vi "RT Main.vi"() -> ()   [LabVIEW 2018]
doc: "The myRIO Custom FPGA Project template acquires button data from the onboard button and displays the button value on a Boolean indicator. The SYS.RDY indicator shows the FPGA status."
uses:
  <vilib>/Stratom, Inc/X-CAN for myRIO (API)/X-CAN Class/Type Definitions/CANFrame.ctl
  <vilib>/Stratom, Inc/X-Modules for myRIO/Type Defs/MXPChannel.ctl
  <vilib>/Stratom, Inc/X-CAN for myRIO (API)/X-CAN Class/Type Definitions/CAN_Speed.ctl
  <vilib>/Platform/TimedLoop/XDataNode/timing_clust.ctl
  <vilib>/Platform/TimedLoop/XDataNode/nitl_modes.ctl
  <vilib>/Platform/TimedLoop/XDataNode/wakeup.ctl
  <vilib>/myRIO/Instrument Drivers/Onboard IO/I2C/typedefs/I2C User Configuration.ctl
  <vilib>/myRIO/Instrument Drivers/Onboard IO/I2C/typedefs/I2C Transfer Rate.ctl
  <vilib>/myRIO/Instrument Drivers/Onboard IO/I2C/typedefs/I2C Reference.ctl
  <vilib>/myRIO/Common/Instrument Driver Framework/Utilities/typedefs/myRIO Generic Hardware Reference.ctl
  <vilib>/myRIO/Common/Instrument Driver Framework/Utilities/typedefs/Hardware Version Enum.ctl
  <vilib>/myRIO/Common/Instrument Driver Framework/Utilities/typedefs/myRIO v1.0 Reference.ctl
  <vilib>/myRIO/Common/Instrument Driver Framework/Utilities/typedefs/Generic FPGA Reference.ctl
  <vilib>/myRIO/Common/Instrument Driver Framework/myRIO v1.0/I2C/typedefs/I2C Channels Enum.ctl
  <vilib>/myRIO/Instrument Drivers/Onboard IO/I2C/typedefs/I2C Configuration.ctl
  <vilib>/userdefined/High Color/nirio_resource_hc.ctl
  <vilib>/myRIO/Instrument Drivers/Onboard IO/AI/typedefs/AI Reference.ctl
  <vilib>/myRIO/Common/Instrument Driver Framework/myRIO v1.0/AI/typedefs/AI Channels List.ctl
  <vilib>/myRIO/Common/Instrument Driver Framework/myRIO v1.0/AI/typedefs/AI Channels Enum.ctl
  <vilib>/myRIO/Common/Instrument Driver Framework/Utilities/typedefs/Analog Scaling Constants List.ctl
  <vilib>/myRIO/Common/Instrument Driver Framework/Utilities/typedefs/Analog Scaling Constants.ctl
  <vilib>/myRIO/Instrument Drivers/Onboard IO/DIO/typedefs/DIO Reference.ctl
  <vilib>/myRIO/Common/Instrument Driver Framework/myRIO v1.0/DIO/typedefs/DIO Channels List.ctl
  <vilib>/myRIO/Common/Instrument Driver Framework/myRIO v1.0/DIO/typedefs/DIO Channels Enum.ctl
  <vilib>/imath/engines/lvmath/Plug In/_Char/NIMS_CH_character datatype.ctl
  <vilib>/myRIO/Instrument Drivers/Onboard IO/AO/typedefs/AO Reference.ctl
  <vilib>/myRIO/Common/Instrument Driver Framework/myRIO v1.0/AO/typedefs/AO Channels List.ctl
  <vilib>/myRIO/Common/Instrument Driver Framework/myRIO v1.0/AO/typedefs/AO Channels Enum.ctl
  <vilib>/myRIO/Common/Instrument Driver Framework/Utilities/vis/Is FPGA Ref Available.vi
  <vilib>/myRIO/Common/Instrument Driver Framework/myRIO v1.0/I2C/vis/myRIO v1.1 Open I2C.vi
  <vilib>/myRIO/Instrument Drivers/Onboard IO/I2C/vis/Configure.vi
  <vilib>/myRIO/Instrument Drivers/Onboard IO/I2C/vis/Write Read.vi
  <vilib>/myRIO/Common/Instrument Driver Framework/myRIO v1.0/AI/vis/myRIO v1.1 Open AI.vi
  <vilib>/myRIO/Instrument Drivers/Onboard IO/AI/vis/Read.vi
  <vilib>/myRIO/Common/Instrument Driver Framework/myRIO v1.0/DIO/vis/myRIO v1.1 Open DIO.vi
  <vilib>/myRIO/Instrument Drivers/Onboard IO/DIO/vis/Write.vi
  <vilib>/myRIO/Common/Instrument Driver Framework/myRIO v1.0/AO/vis/myRIO v1.1 Open AO.vi
  <vilib>/myRIO/Instrument Drivers/Onboard IO/AO/vis/Write.vi
  <vilib>/myRIO/Instrument Drivers/Onboard IO/DIO/vis/Read.vi
  <vilib>/myRIO/Common/Instrument Driver Framework/Utilities/vis/Validate Channels.vi
  <vilib>/myRIO/Common/Instrument Driver Framework/myRIO v1.0/I2C/vis/myRIO v1.0 Reserve I2C.vi
  <vilib>/myRIO/Common/Instrument Driver Framework/myRIO v1.0/AI/vis/myRIO v1.0 Reserve AI.vi
  <vilib>/myRIO/Common/Instrument Driver Framework/myRIO v1.0/DIO/vis/myRIO v1.0 Reserve DIO.vi
  <vilib>/myRIO/Common/Instrument Driver Framework/myRIO v1.0/AO/vis/myRIO v1.0 Reserve AO.vi
  <vilib>/myRIO/Common/Instrument Driver Framework/myRIO v1.0/I2C/vis/myRIO v1.0 Build MUX Configuration I2C.vi
  <vilib>/myRIO/Common/Instrument Driver Framework/myRIO v1.0/Resource Manager/vis/myRIO v1.0 Reserve Channel List.vi
  <vilib>/myRIO/Common/Instrument Driver Framework/myRIO v1.0/AI/vis/myRIO v1.0 Build MUX Configuration AI.vi
  <vilib>/myRIO/Common/Instrument Driver Framework/myRIO v1.0/DIO/vis/myRIO v1.0 Build MUX Configuration DIO.vi
  <vilib>/myRIO/Common/Instrument Driver Framework/myRIO v1.0/AO/vis/myRIO v1.0 Build MUX Configuration AO.vi
  <vilib>/myRIO/Common/Instrument Driver Framework/myRIO v1.0/Resource Manager/vis/myRIO v1.0 Create Configuration List.vi
  <vilib>/myRIO/Common/Instrument Driver Framework/myRIO v1.0/Resource Manager/vis/myRIO v1.0 Reserve Channel.vi
  <vilib>/myRIO/Common/Instrument Driver Framework/myRIO v1.0/Resource Manager/vis/myRIO v1.0 Unreserve Channel.vi
  <vilib>/myRIO/Common/Instrument Driver Framework/myRIO v1.0/Resource Manager/vis/myRIO v1.0 Build Mutex Name.vi
  <vilib>/functionblocks/Counter/Pulse Timer/Pulse Timer.vi
  <vilib>/Utility/VariantDataType/GetNumericInfo.vi
  <vilib>/Utility/error.llb/Error Cluster From Error Code.vi
  <vilib>/myRIO/Common/Instrument Driver Framework/myRIO v1.0/myRIO v1.1 Open.vi
  <vilib>/myRIO/Common/Instrument Driver Framework/Utilities/vis/IO Manager.vi
  <vilib>/myRIO/Common/Instrument Driver Framework/Utilities/vis/Configuration Manager.vi
  <vilib>/myRIO/Common/Instrument Driver Framework/myRIO v1.0/Resource Manager/vis/myRIO v1.0 Configure IO.vi
  <vilib>/myRIO/Common/Instrument Driver Framework/myRIO v1.0/myRIO v1.0 Close.vi
  <vilib>/myRIO/Common/Instrument Driver Framework/myRIO v1.0/DIO/vis/myRIO v1.0 Read DIO.vi
  <vilib>/myRIO/Common/Instrument Driver Framework/myRIO v1.0/DIO/vis/myRIO v1.0 Write DIO.vi
  <vilib>/myRIO/Common/Instrument Driver Framework/myRIO v1.0/AI/vis/myRIO v1.0 Get Scaling Constants AI.vi
  <vilib>/myRIO/Common/Instrument Driver Framework/myRIO v1.0/AI/vis/myRIO v1.0 Read AI.vi
  <vilib>/functionblocks/Bistables/SR Bistable/SR Bistable.vi
  <vilib>/myRIO/Common/Instrument Driver Framework/myRIO v1.0/AO/vis/myRIO v1.0 Get Scaling Constants AO.vi
  <vilib>/myRIO/Common/Instrument Driver Framework/myRIO v1.0/AO/vis/myRIO v1.0 Write AO.vi
  <vilib>/imath/engines/lvmath2/RunTimeEngine/Managers/WorkSpace/UID Generator.vi
  <vilib>/imath/engines/lvmath/Plug In/_Char/NIMS_CH_Character 1D to U8 1D.vi
  <vilib>/imath/engines/lvmath2/RunTimeEngine/BuiltInFunctions/double/NIMS_double.vi
  <instcachedir>/0/NIMS_double_34E32F64C2B04A25A042F4CA881A0A41.lvgen/NIMS_double_34E32F64C2B04A25A042F4CA881A0A41_002.vi
  <vilib>/imath/engines/lvmath2/RunTimeEngine/RunTimeType/NIMS_RunTimeType_From StrictType (excl LVString).vi
  <instcachedir>/0/NIMS_RunTimeType_From StrictType (excl LVString)_E7E34A65C99947108168652BAD14964D.lvgen/NIMS_RunTimeType_From StrictType (excl LVString)_E7E34A65C99947108168652BAD14964D_000.vi
  <vilib>/imath/engines/lvmath2/RunTimeEngine/LocalVariableDefStatement/MC_LocalVariableDefStatement_Display.vi
  <vilib>/imath/engines/lvmath2/RunTimeEngine/BuiltInFunctions/min/2 inputs/NIMS_min(RG,RG)-no size check.vi
  <instcachedir>/0/NIMS_min(RG,RG)-no size check_7F67BAB91AFC452D9517D2EA1C8F5F88.lvgen/NIMS_min(RG,RG)-no size check_7F67BAB91AFC452D9517D2EA1C8F5F88_001.vi
  <vilib>/imath/engines/lvmath2/RunTimeEngine/Managers/SymbolTable/Clear UID.vi
  <vilib>/imath/engines/lvmath2/RunTimeEngine/NodeEndStatement/NIMS_NodeEndStatement_Output.vi
  <instcachedir>/0/NIMS_NodeEndStatement_Output_53EC0D466D134D7ABD903AC30B43404B.lvgen/NIMS_NodeEndStatement_Output_53EC0D466D134D7ABD903AC30B43404B_001.vi
  <vilib>/imath/engines/lvmath2/RunTimeEngine/ErrorHandling/NIMS_Finalize Error.vi
  <vilib>/myRIO/Common/Instrument Driver Framework/myRIO v1.0/I2C/vis/myRIO v1.0 Configure I2C.vi
  <vilib>/myRIO/Common/Instrument Driver Framework/myRIO v1.0/I2C/vis/myRIO v1.0 Write I2C.vi
  <vilib>/myRIO/Common/Instrument Driver Framework/myRIO v1.0/I2C/vis/myRIO v1.0 Read I2C.vi
  <vilib>/Platform/TimedLoop/XDataNode/XDataNode.xnode
  <vilib>/functionblocks/FB Core/FB Core.xnode
  <vilib>/myRIO/Express VI/Onboard IO/DI/DI Express VI.xnode
  <vilib>/myRIO/Instrument Drivers/Onboard IO/DIO/vis/myRIO DIO Open.xnode
  <vilib>/myRIO/Express VI/Onboard IO/DO/DO Express VI.xnode
  <vilib>/myRIO/Express VI/Onboard IO/AI/AI Express VI.xnode
  <vilib>/myRIO/Instrument Drivers/Onboard IO/AI/vis/myRIO AI Open.xnode
  <vilib>/myRIO/Express VI/Onboard IO/AO/AO Express VI.xnode
  <vilib>/myRIO/Instrument Drivers/Onboard IO/AO/vis/myRIO AO Open.xnode
  <vilib>/myRIO/Express VI/Onboard Devices/LED/LED Express VI.xnode
  <vilib>/myRIO/Express VI/Onboard IO/I2C/I2C Express VI.xnode
  <vilib>/myRIO/Instrument Drivers/Onboard IO/I2C/vis/myRIO I2C Open.xnode
  <vilib>/myRIO/Instrument Drivers/Onboard IO/DIO/DIO.lvlib
  <vilib>/functionblocks/NI_FunctionBlock Libraries.lvlib
  <vilib>/myRIO/Instrument Drivers/Onboard IO/AI/AI.lvlib
  <vilib>/Platform/TimedLoop/XDataNode/XDNodeRunTimeDep.lvlib
  <vilib>/myRIO/Instrument Drivers/Onboard IO/AO/AO.lvlib
  <vilib>/myRIO/Instrument Drivers/Onboard IO/I2C/I2C.lvlib
  <vilib>/Stratom, Inc/X-CAN for myRIO (API)/X-CAN Class/X-CAN.lvclass
  <vilib>/imath/engines/lvmath2/RunTimeEngine/Managers/SymbolTable/NIMS_WorkSpace.lvlib
panel:
  in  "Stop Button":bool
  out "LEDs":bool[](array[boolean])
  out "Data Ready?":bool
  out "CAN Frame":T1 {"payload" format="%x"; "timestamp" format="%<%I:%M:%S%8u %p\n%x>T"; "identifier" format="%x"}
  out "Current Device":dbl format="%.2f"
  out "Current 200pc":dbl format="%.2f"
  out "Current Actual":dbl format="%.2f"
  out "speed actual":dbl format="%.2f"
  out "Motor RPM":dbl(knob) scale=0.0..5700.0
  out "Actual Bamocar Current":dbl
  out "IGBT temp":dbl format="%.2f"
  out "I Filter":dbl format="%.2f"
  out "Motor Temp":dbl format="%.2f"
  out "Highest Cell Volt":dbl
  out "Lowest Cell Volt":dbl
  out "Highest Temp":u16
  out "Lowest Temp":u16
  out "Current Sensor":u16
  out "Accumulator Voltage":u16
  out "WS FL":dbl
  out "WS FR":dbl
  out "WS RL":dbl
  out "WS RR":dbl
  out "Accelerometer x":dbl
  out "Accelerometer y":dbl
  out "Accelerometer z":dbl
  out "Torque Constant":dbl
  out "Speed Rpm max int":dbl format="%.2f"
  out "Array":u8[](array[numeric])
  out "loop counter":i32
  out "Bytes Read":u8[](array[numeric])
  out "Slave Address (7-bit)":u8=4
  out "Byte Count":u32=168
  out "high byte":u8
  out "low byte":u8
  out "Values":dbl[](array[numeric])
  out "Stack 1 vol":dbl[](array[numeric])
  out "Stack 2 vol":dbl[](array[numeric])
  out "Stack 3 vol":dbl[](array[numeric])
  out "Stack 4 vol":dbl[](array[numeric])
  out "Stack 5 vol":dbl[](array[numeric])
  out "Stack 1 temp":dbl[](array[numeric])
  out "Stack 2 temp":dbl[](array[numeric])
  out "Stack 3 temp":dbl[](array[numeric])
  out "Stack 4 temp":dbl[](array[numeric])
  out "Stack 5 temp":dbl[](array[numeric])
  out "AMS current":dbl[](array[numeric])
  out "Coulomb Counting":dbl[](array[numeric])
  in  "stop":bool
  out "APPS1 (V) Input (B/AI0 (Pin 3))":dbl
  out "APPS2 Scaled Up (V)":dbl
  out "APPS1 Scaled Up (V)":dbl
  out "APPS2 (V) Input (B/AI1 (Pin 5))":dbl
  out "APPS fault":bool
  out "APPS2 %":dbl
  out "APPS1 %":dbl
  out "APPS Output (V)":dbl
  out "APPS output %":dbl
  out "Accelaration":dbl(knob) scale=0.0..100.0
  out "APPS1":dbl(knob) scale=0.0..100.0
  out "APPS2":dbl(knob) scale=0.0..100.0
  out "APPS pedal travel %":dbl
  out "RTD Status LED":bool
  out "RFE Indicator":bool
  out "AIR + Boolean":bool
  out "AIR +(A9)":dbl
  out "RTD Button":bool
  out "RTD Brake":bool
  out "EN Indicator":bool
  out "RTD Buzzer":bool
  in  "Buzzer test":bool
  in  "RTD Brake Test":bool
  in  "RFE  Test":bool
  in  "EN Test":bool
  out "Pump out":bool
  in  "Pump Test":bool
  out "Bamocar Temp Threshold":bool
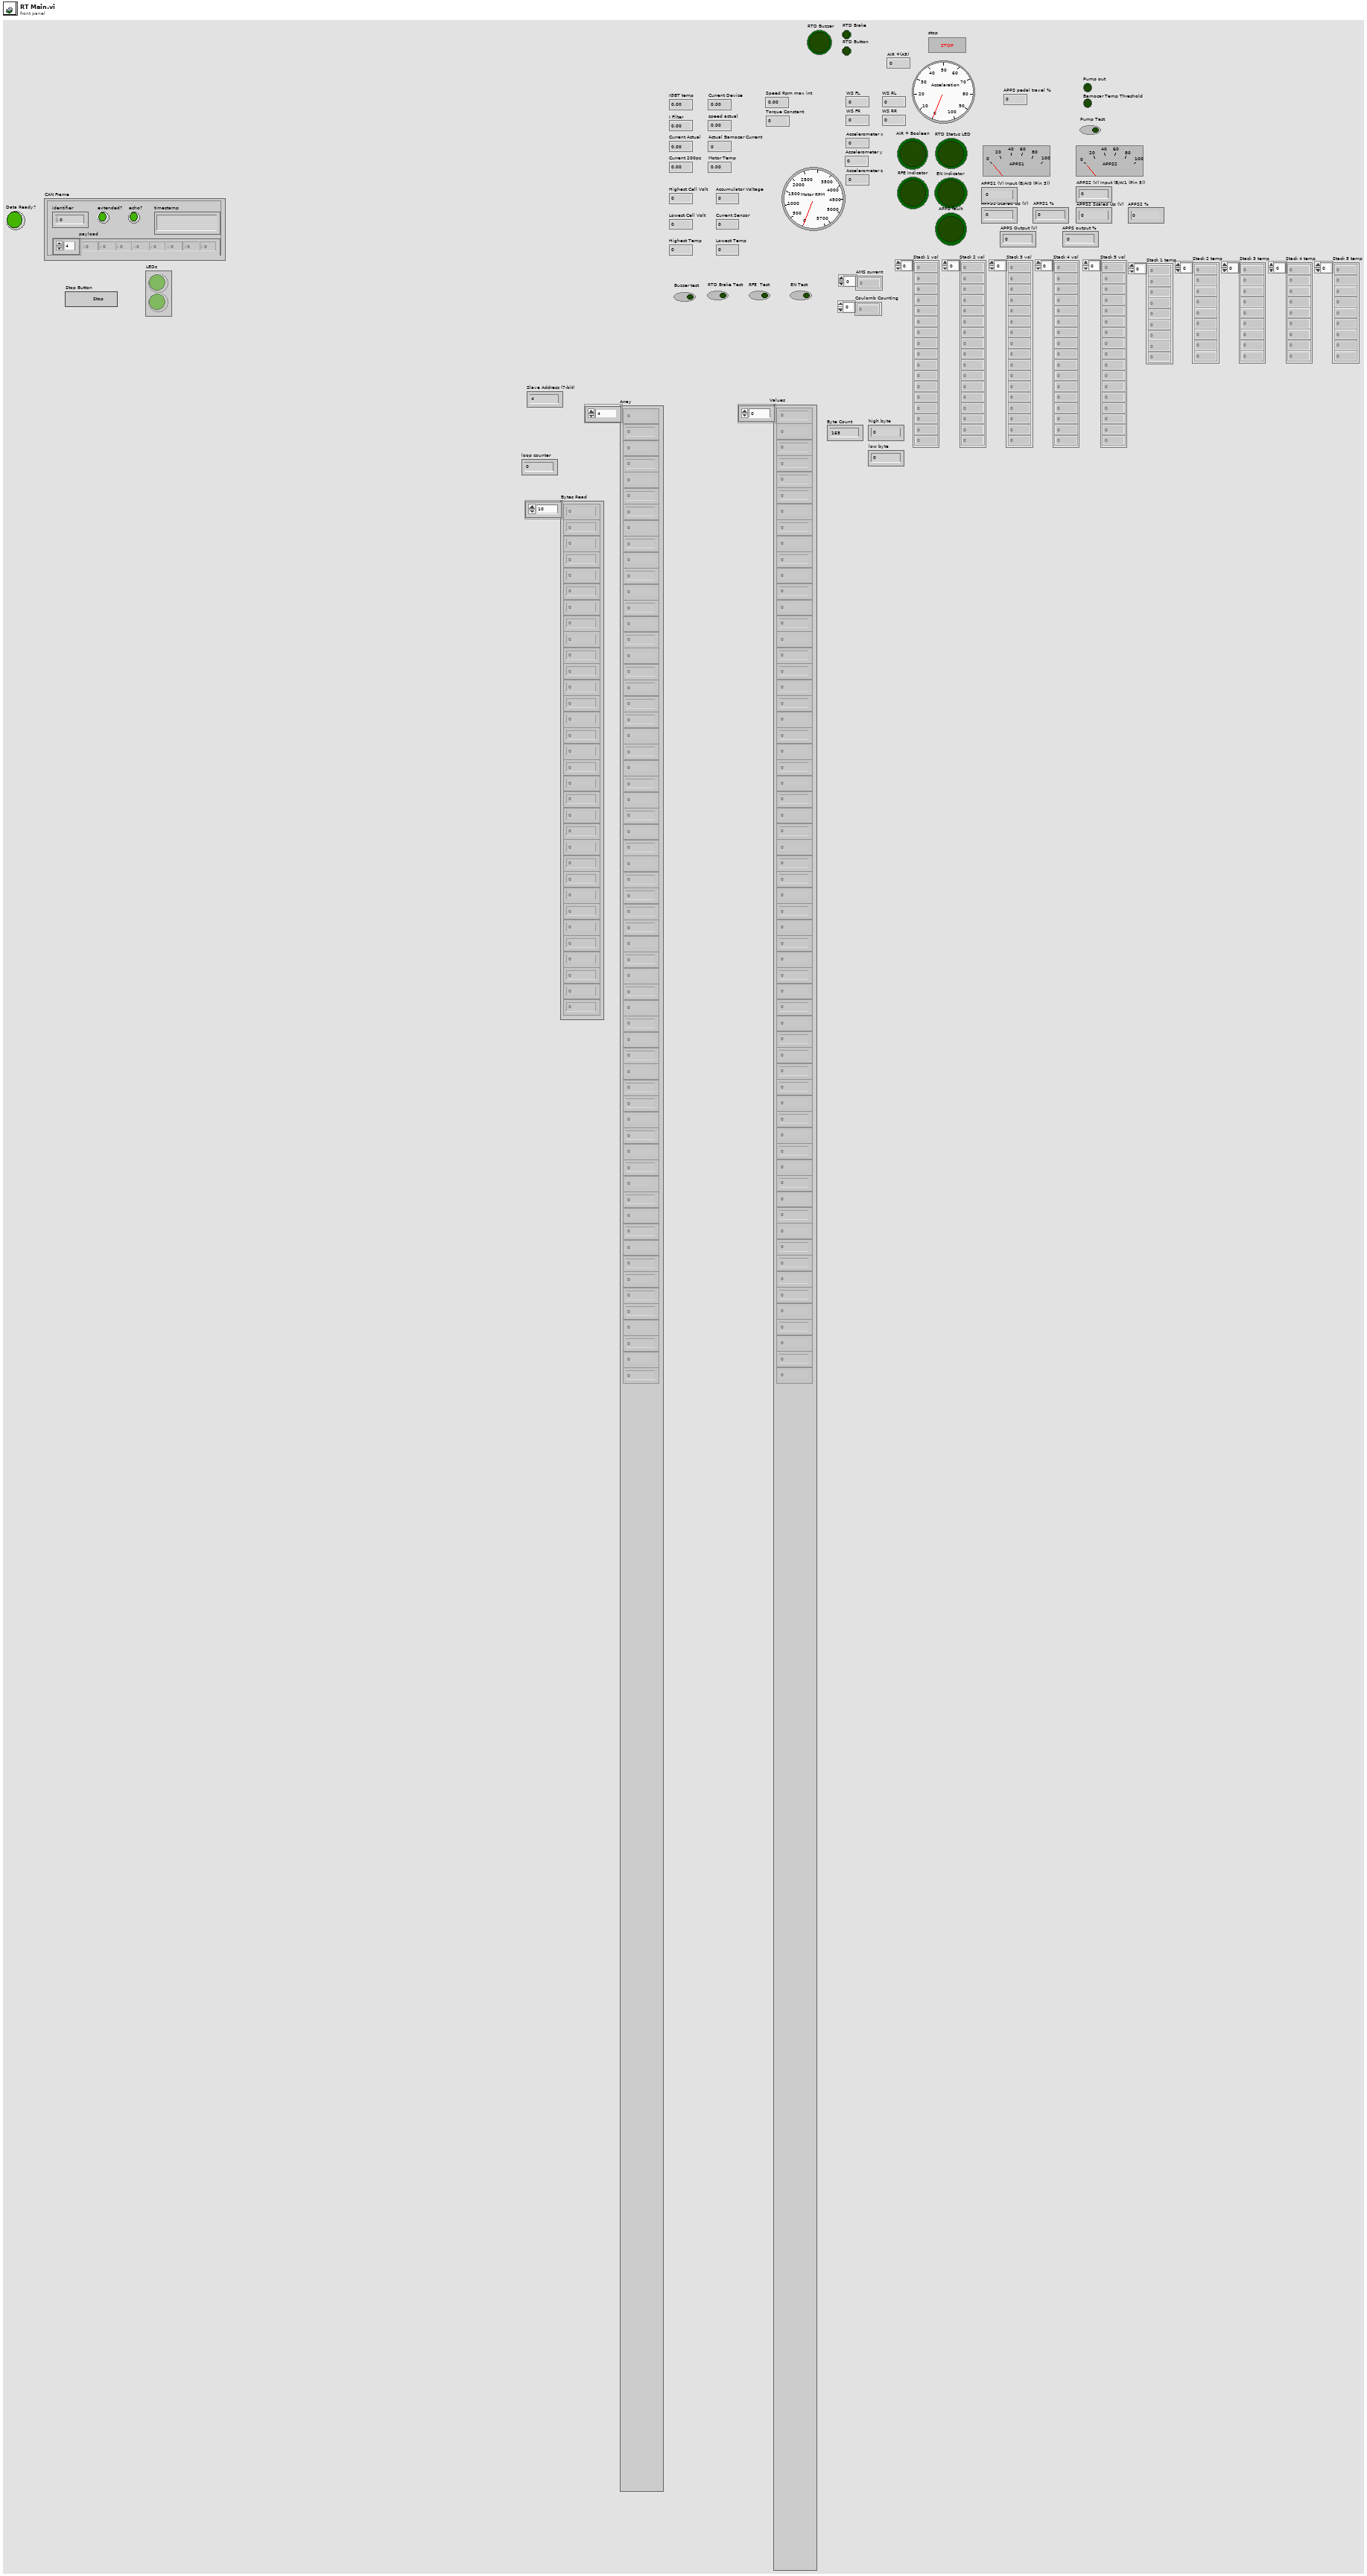
[diagram p1: front panel]
types:
  T1 = typedef "X-CAN.lvclass/CANFrame.ctl" = cluster{"identifier":u32, "extended?":bool, "echo?":bool, "payload":u8[], "timestamp":timestamp}
  T2 = typedef "X-CAN.lvclass/CAN_Speed.ctl" = u8
  T3 = typedef "MXPChannel.ctl" = enum16{"A/MXP", "B/MXP"}
  T4 = typedef "XDNodeRunTimeDep.lvlib/timing_clust.ctl" = cluster{"Expected End [f-1]":u64, "Actual End [f-1]":u64, "Finished Late? [f-1]":bool, "Expected End [i-1]":u64, "Actual End [i-1]":u64, "Finished Late? [i-1]":bool, "Expected Start [i]":u64, "Actual Start [i]":u64, "Expected Start [f]":u64, "Actual Start [f]":u64, "Source Name":string, "Structure Name":string, "Period":i64, "Deadline":i64, "Offset":i64, "Start":i64, "Priority":i32, "Timeout":i32, "Mode":T5, "Wakeup Reason":T6, "Error":errorcluster, "Source Type":string, "Secondary Source Type":string, "Global End Time":u64, "Global Start Time":u64, "Frame Duration":u64, "Iteration Duration":u64, "Assigned CPU":i32, "I/O Scan Engine Mode":u32}
  T5 = typedef "XDNodeRunTimeDep.lvlib/nitl_modes.ctl" = enum32{"No Change", "Process missed periods, maintain original phase", "Discard missed periods, maintain original phase", "Process missed periods, ignore original phase", "Discard missed periods, ignore original phase"}
  T6 = typedef "XDNodeRunTimeDep.lvlib/wakeup.ctl" = enum32{"Normal", "Aborted", "Asynchronous wakeup", "Timing source error", "Timed loop error", "Timeout"}
  T7 = typedef "NIMS_CH_character datatype.ctl" = cluster{"Numeric":u8}
  T8 = typedef "DIO.lvlib/DIO Reference.ctl" = cluster{"myRIO Reference":T9, "DIO Channels List":T13}
  T9 = typedef "myRIO Generic Hardware Reference.ctl" = cluster{"myRIO Model":T10, "myRIO Hardware Reference":T11}
  T10 = typedef "Hardware Version Enum.ctl" = enum16{"Unknown", "myRIO-1900", "myRIO-1950", "roboRIO", "NI ELVIS RIO CM", "ELVIS III"}
  T11 = typedef "myRIO v1.0 Reference.ctl" = cluster{"Generic FPGA Reference":T12, "Allow multiple opens":bool}
  T12 = typedef "Generic FPGA Reference.ctl" = refnum<k20>
  T13 = typedef "DIO Channels List.ctl" = T14[]
  T14 = typedef "DIO Channels Enum.ctl" = enum16{"Not Connected", "C/DIO0", "C/DIO1", "C/DIO2", "C/DIO3", "C/DIO4", "C/DIO5", "C/DIO6", "C/DIO7", "A/DIO0", "A/DIO1", "A/DIO2", "A/DIO3", "A/DIO4", "A/DIO5", "A/DIO6", "A/DIO7", "A/DIO8", "A/DIO9", "A/DIO10", "A/DIO11", "A/DIO12", "A/DIO13", "A/DIO14", "A/DIO15", "A/DIO16", "A/DIO17", "A/DIO18", "A/DIO19", "B/DIO0", "B/DIO1", "B/DIO2", "B/DIO3", "B/DIO4", "B/DIO5", "B/DIO6", "B/DIO7", "B/DIO8", "B/DIO9", "B/DIO10", "B/DIO11", "B/DIO12", "B/DIO13", "B/DIO14", "B/DIO15", "B/DIO16", "B/DIO17", "B/DIO18", "B/DIO19", "LED0", "LED1", "LED2", "LED3", "Button0", "DIO/DIO0", "DIO/DIO1", "DIO/DIO2", "DIO/DIO3", "DIO/DIO4", "DIO/DIO5", "DIO/DIO6", "DIO/DIO7", "DIO/DIO8", "DIO/DIO9", "SPI/CS0", "SPI/CS1", "SPI/CS2", "SPI/CS3", "LED RADIO (Green)", "LED RADIO (Red)", "LED COMM (Green)", "LED COMM (Red)", "LED MODE (Green)", "LED MODE (Red)"}
  T15 = typedef "nirio_resource_hc.ctl" = tag
  T16 = typedef "AO.lvlib/AO Reference.ctl" = cluster{"myRIO Reference":T9, "AO Channel List":T17, "AO Scaling Constant List":T19}
  T17 = typedef "AO Channels List.ctl" = T18[]
  T18 = typedef "AO Channels Enum.ctl" = enum16{"Not Connected", "AudioOut/Left", "AudioOut/Right", "C/AO0", "C/AO1", "A/AO0", "A/AO1", "B/AO0", "B/AO1"}
  T19 = typedef "Analog Scaling Constants List.ctl" = T20[]
  T20 = typedef "Analog Scaling Constants.ctl" = cluster{"LSB Weight (Volts)":dbl, "Offset (Volts)":dbl, "Signed?":bool}
  T21 = typedef "AI.lvlib/AI Reference.ctl" = cluster{"myRIO Reference":T9, "AI Channels List":T22, "AI Scaling Constants List":T19}
  T22 = typedef "AI Channels List.ctl" = T23[]
  T23 = typedef "AI Channels Enum.ctl" = enum16{"Not Connected", "AudioIn/Left", "AudioIn/Right", "C/AI0", "C/AI1", "A/AI0", "A/AI1", "A/AI2", "A/AI3", "A/AI4", "A/AI5", "A/AI6", "A/AI7", "B/AI0", "B/AI1", "B/AI2", "B/AI3", "B/AI4", "B/AI5", "B/AI6", "B/AI7", "AI/AI0", "AI/AI1", "AI/AI2", "AI/AI3", "A/AI0 (DIFF)", "A/AI1 (DIFF)", "A/AI2 (DIFF)", "A/AI3 (DIFF)", "B/AI0 (DIFF)", "B/AI1 (DIFF)", "B/AI2 (DIFF)", "B/AI3 (DIFF)"}
  T24 = typedef "I2C.lvlib/I2C Reference.ctl" = cluster{"myRIO Reference":T9, "I2C Channels Enum":T25, "I2C Configuration":T26}
  T25 = typedef "I2C Channels Enum.ctl" = enum16{"Not Connected", "A/I2C", "B/I2C", "I2C/I2C"}
  T26 = typedef "I2C.lvlib/I2C Configuration.ctl" = cluster{"I2C Transfer Rate":T27}
  T27 = typedef "I2C.lvlib/I2C Transfer Rate.ctl" = enum16{"Standard mode (100 kbps)", "Fast mode (400 kbps)"}
  T28 = typedef "I2C.lvlib/I2C User Configuration.ctl" = cluster{"I2C Transfer Rate":T27}
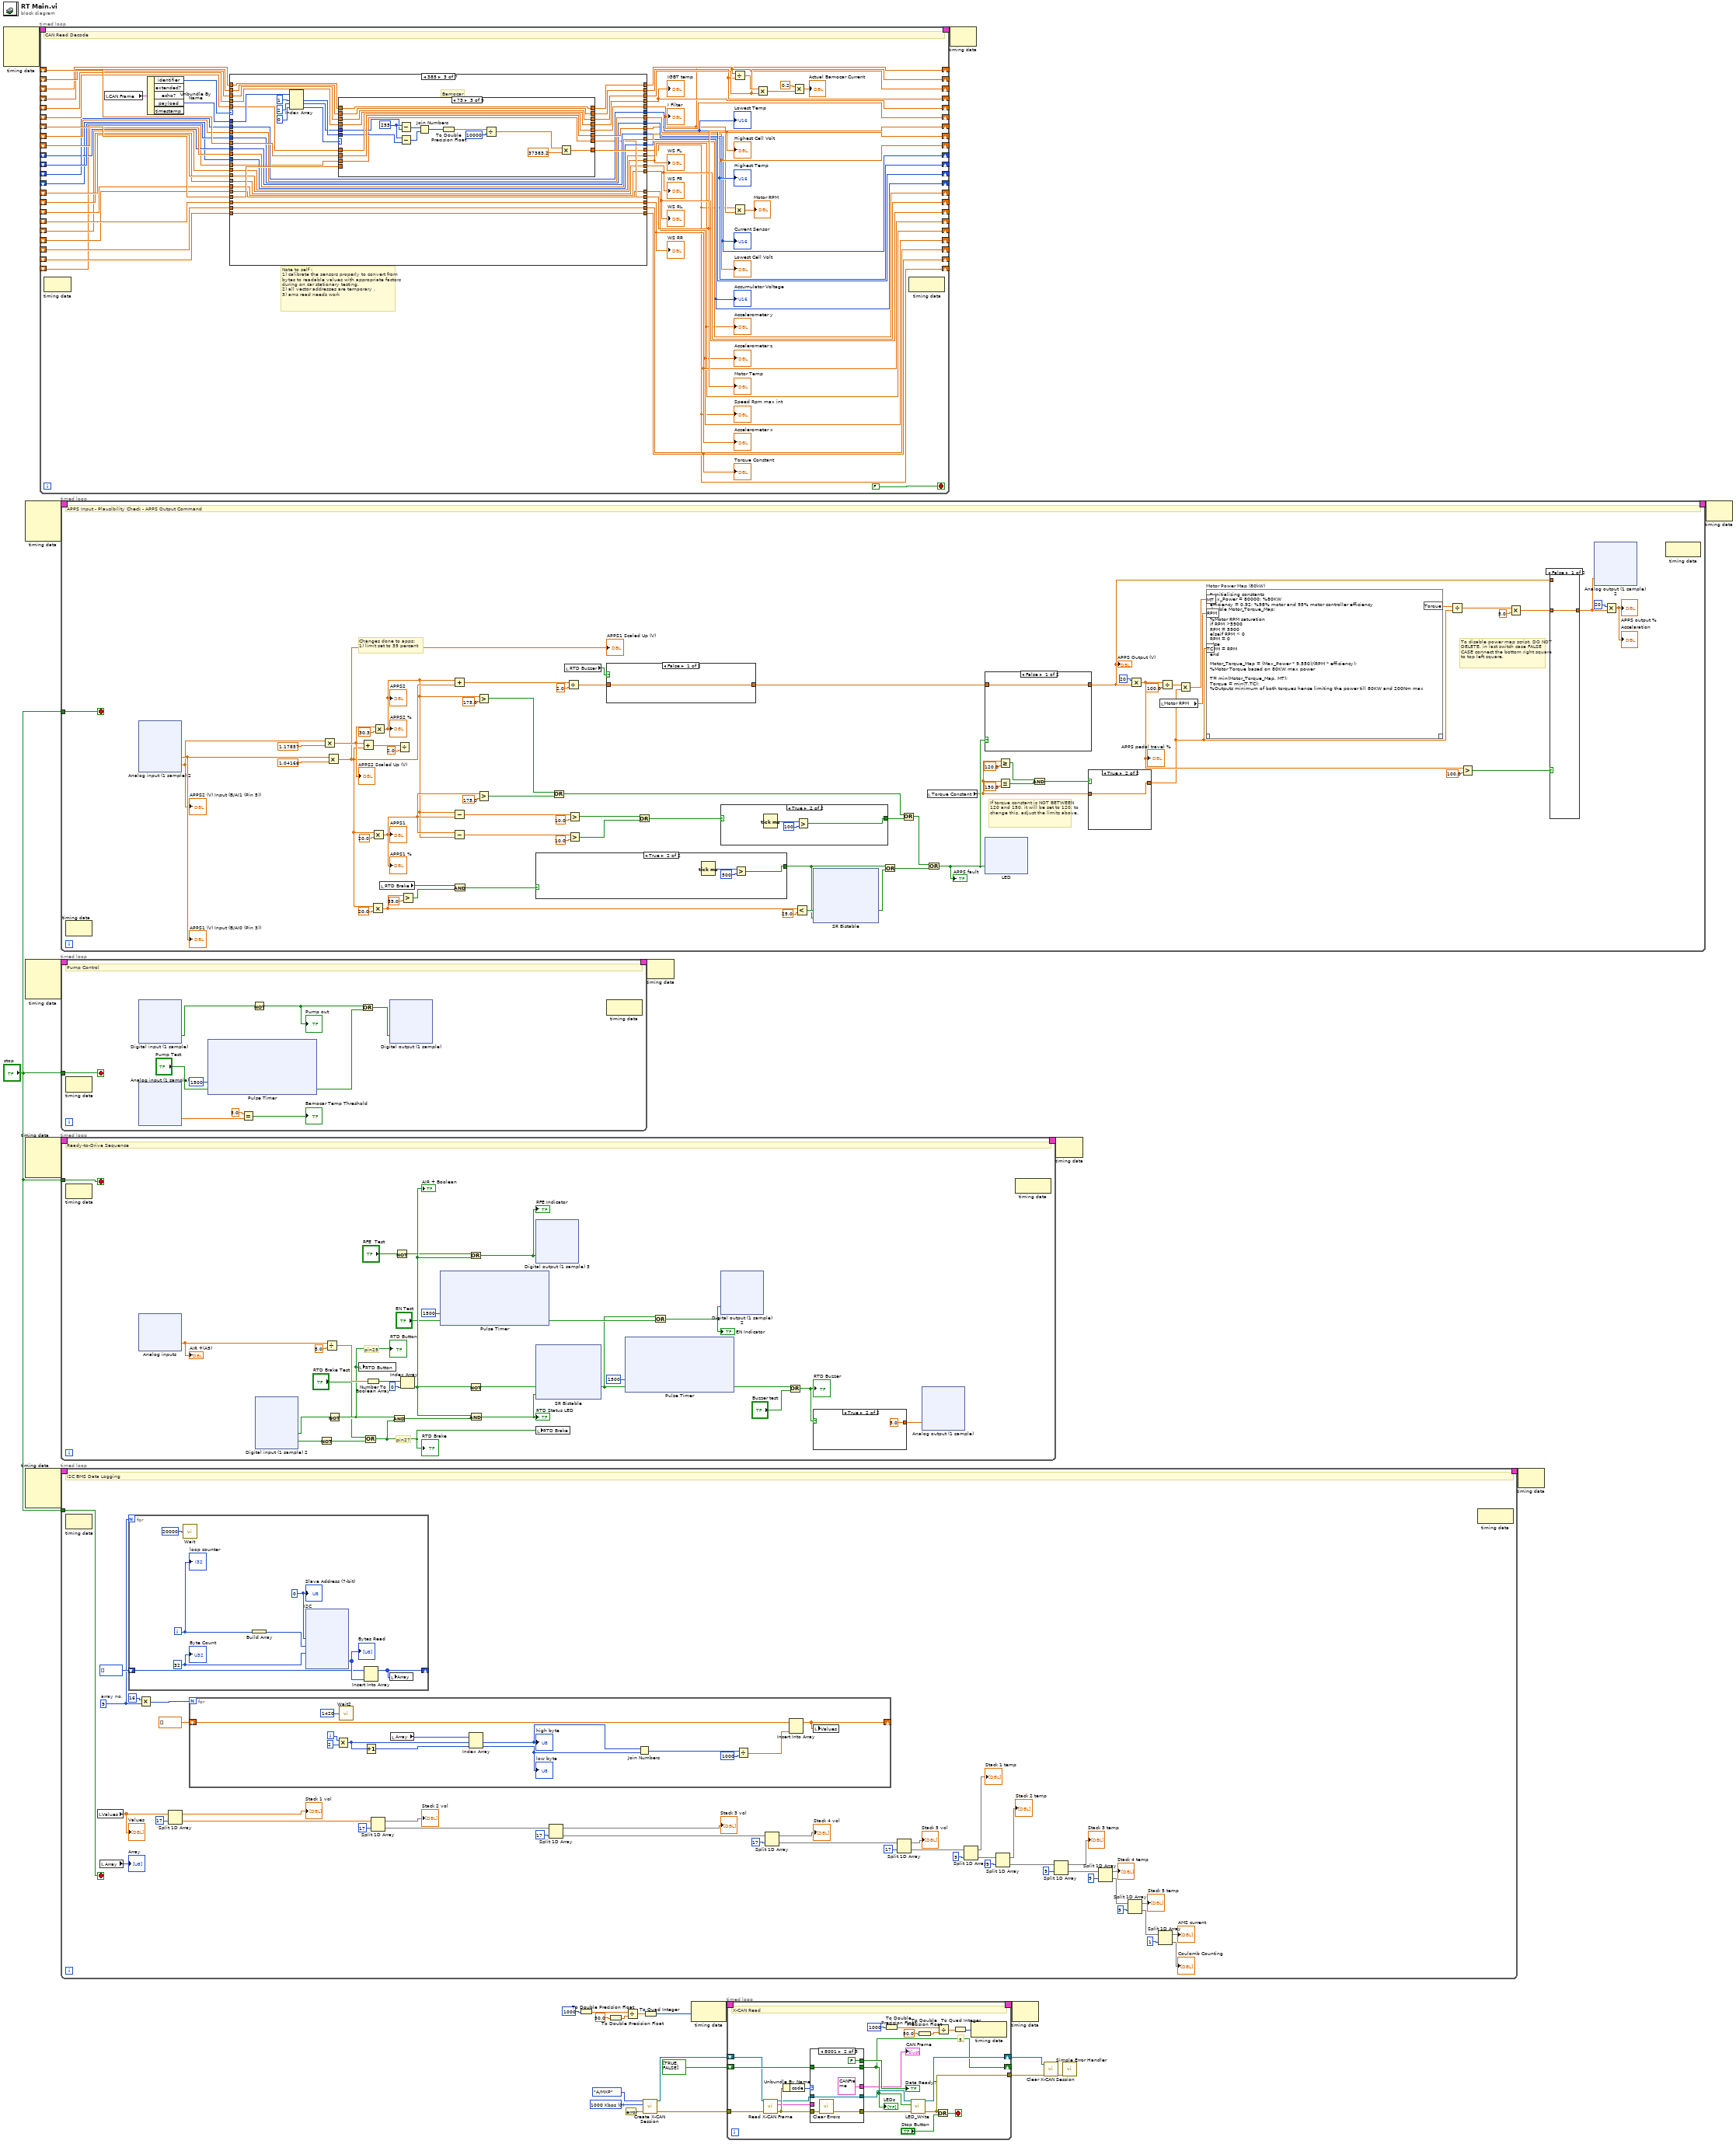
[diagram p0: block diagram]
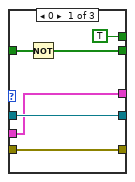
[diagram p2: hidden frame]
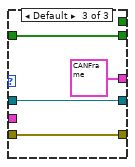
[diagram p3: hidden frame]
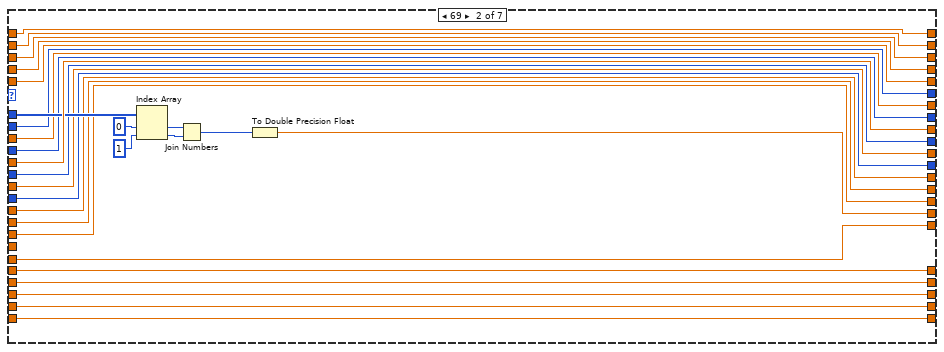
[diagram p5: hidden frame]
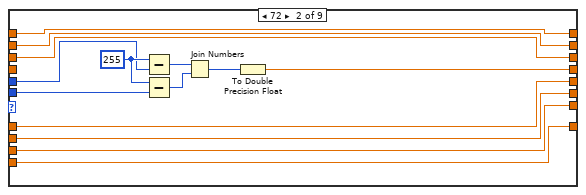
[diagram p7: hidden frame]
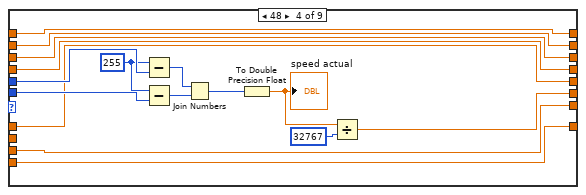
[diagram p8: hidden frame]
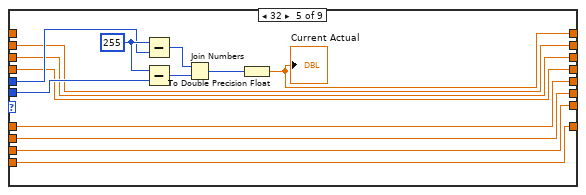
[diagram p9: hidden frame]
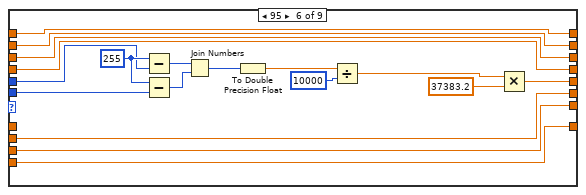
[diagram p10: hidden frame]
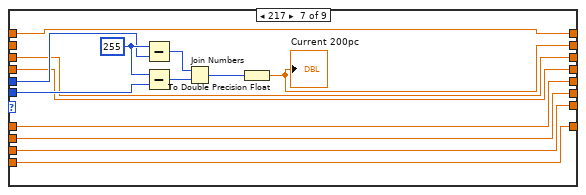
[diagram p11: hidden frame]
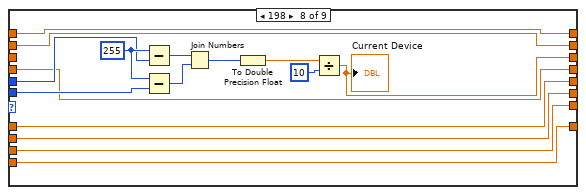
[diagram p12: hidden frame]
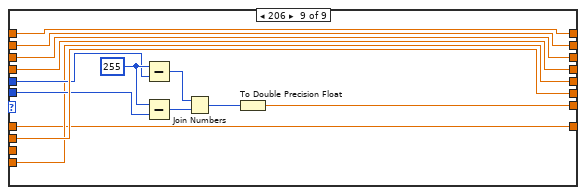
[diagram p13: hidden frame]
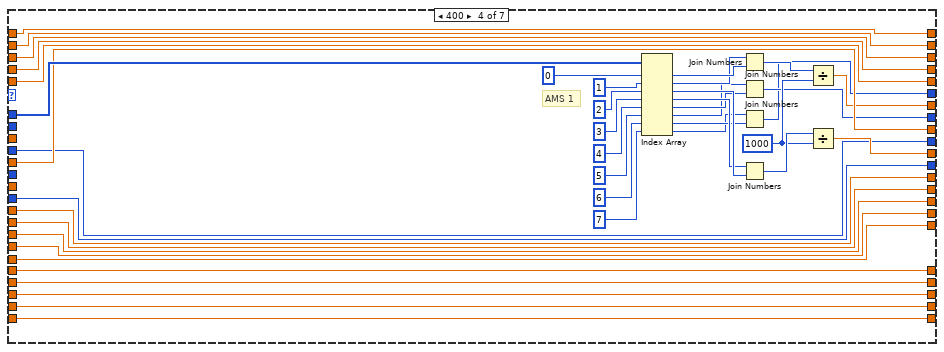
[diagram p14: hidden frame]
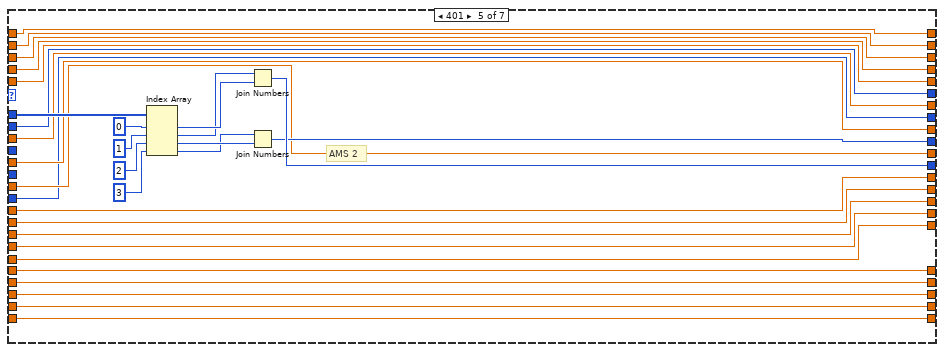
[diagram p15: hidden frame]
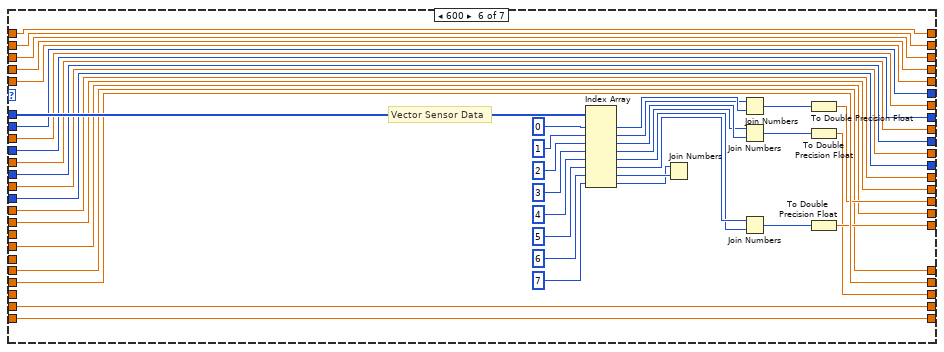
[diagram p16: hidden frame]
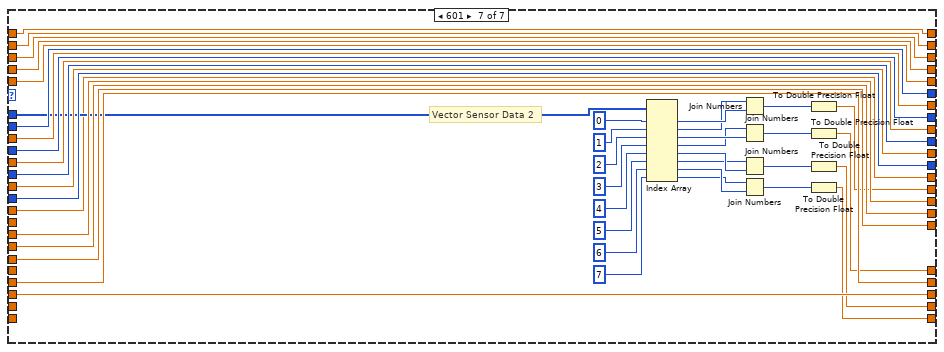
[diagram p17: hidden frame]
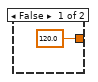
[diagram p18: hidden frame]
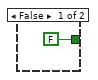
[diagram p19: hidden frame]
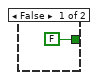
[diagram p20: hidden frame]
diagram:
  w4 = T2 0 items=["125 Kbps"=7, "250 Kbps"=3, "500 Kbps"=1, "1000 Kbps"=0, "95.238 Kbps"=6] ("CAN Speed [Kbps]")
  n1 = node-c288() -> (w20:T4)  [unwired: 4 in]
  n2 = node-c288() -> (w24:T4)  [unwired: 4 in]
  n3 = node-c288() -> (w28:T4)  [unwired: 4 in]
  n4 = node-c288() -> (w26:T4)  [unwired: 4 in]
  n5 = node-c288() -> (w22:T4)  [unwired: 4 in]
  n6 = timed-loop {
    shift-right: [w32] -> _
    shift-left: _ -> [w78]
    shift-right: [w71] -> _
    shift-left: _ -> [w67]
    shift-right: [w72] -> _
    shift-left: _ -> [w69]
    shift-right: [w70] -> _
    shift-left: _ -> [w68]
    shift-right: [w66] -> _
    shift-left: _ -> [w65]
    shift-right: [w64] -> _
    shift-left: _ -> [w63]
    shift-right: [w62] -> _
    shift-left: _ -> [w61]
    shift-right: [w57] -> _
    shift-left: _ -> [w56]
    shift-right: [w58] -> _
    shift-left: _ -> [w55]
    shift-right: [w59] -> _
    shift-left: _ -> [w54]
    shift-right: [w60] -> _
    shift-left: _ -> [w53]
    shift-right: [w50] -> _
    shift-left: _ -> [w51]
    shift-right: [w52] -> _
    shift-left: _ -> [w49]
    shift-right: [w48] -> _
    shift-left: _ -> [w47]
    shift-right: [w44] -> _
    shift-left: _ -> [w41]
    shift-right: [w45] -> _
    shift-left: _ -> [w42]
    shift-right: [w46] -> _
    shift-left: _ -> [w43]
    timing: w20 -> [_]
    timing-out: [_] -> w19
    shift-right: [w40] -> _
    shift-left: _ -> [w36]
    shift-right: [w39] -> _
    shift-left: _ -> [w35]
    shift-right: [w38] -> _
    shift-left: _ -> [w34]
    shift-right: [w37] -> _
    shift-left: _ -> [w33]
    shift-right: [w29] -> _
    shift-left: _ -> [w30]
    stop <- FALSE stop-if-true
    # "Note to self : \n1) calibrate the sensors properly to convert from bytes to readable values with appropriate factors during on car stationary testing.\n2) all vector addresses are temporary .\n3) ams read needs work"
    # "CAN Read Decode"
    n7 = node-c288() -> ()  [unwired: 1 in, 1 out]
    n8 = local read "CAN Frame"() -> (w81:T1)
    n9 = Unbundle By Name(w81) -> ("identifier"=w77:u32, "payload"=w80:u8[])  [unwired: 3 out]
    n10 = case shown="385" w77 {
      tunnel: w80 -> [_ w129 w170 w344 w375 w417 w443]
      tunnel: w78 -> [w105 w132 w164 w324 w364 w400 w460]
      tunnel: [w105 w132 w162 w324 w364 w400 w460] -> w32
      tunnel: [w104 w120 w161 w321 w361 w397 w458] -> w71
      tunnel: [w103 w121 w160 w322 w362 w398 w459] -> w70
      tunnel: [w102 w119 w159 w323 w363 w399 w457] -> w72
      tunnel: w69 -> [w102 w119 w158 w323 w363 w399 w457]
      tunnel: w68 -> [w103 w121 w157 w322 w362 w398 w459]
      tunnel: w67 -> [w104 w120 w156 w321 w361 w397 w458]
      tunnel: [w101 w133 w155 w320 w360 w396 w456] -> w66
      tunnel: w65 -> [w101 w133 w154 w320 w360 w396 w456]
      tunnel: [w100 w131 w153 w319 w359 w395 w455] -> w64
      tunnel: w63 -> [w100 w131 w152 w319 w359 w395 w455]
      tunnel: [w99 w130 w151 w318 w358 w394 w454] -> w62
      tunnel: w61 -> [w99 w130 w150 w318 w358 w394 w454]
      tunnel: [w98 w118 w149 w317 w357 w393 w453] -> w57
      tunnel: [w97 w117 w148 w316 w356 w392 w452] -> w58
      tunnel: [w96 w115 w147 w315 w355 w388 w450] -> w59
      tunnel: [w95 w113 w146 w314 w354 w390 w449] -> w60
      tunnel: w56 -> [w98 w118 w149 _ w357 w393 w453]
      tunnel: w55 -> [w97 w117 w148 _ w356 w392 w452]
      tunnel: w54 -> [w96 w115 w147 w313 _ w388 w450]
      tunnel: w53 -> [w95 w113 w146 _ w354 w390 w449]
      tunnel: [w94 w112 w144 w312 w366 w391 w448] -> w52
      tunnel: w51 -> [w93 w116 w145 _ _ w389 w451]
      tunnel: [w93 w116 w145 w313 w365 w389 w451] -> w50
      tunnel: w49 -> [w94 w112 w144 w312 w355 w391 w448]
      tunnel: [w89 w122 w140 w311 w353 w387 w447] -> w48
      tunnel: [w92 w110 w143 w308 w350 w383 w444] -> w44
      tunnel: [w91 w111 w142 w309 w351 w385 w445] -> w45
      tunnel: [w90 w123 w141 w310 w352 w376 w446] -> w46
      tunnel: w47 -> [w89 w122 w140 w311 w353 _ w447]
      tunnel: w43 -> [w90 _ w141 w310 w352 w376 w446]
      tunnel: w42 -> [w91 w111 w142 w309 w351 _ w445]
      tunnel: w41 -> [w92 w110 w143 w308 w350 _ w444]
      tunnel: [w88 w109 w139 w307 w349 w381 w422] -> w40
      tunnel: [w87 w108 w138 w306 w348 w380 w421] -> w39
      tunnel: [w86 w107 w137 w305 w347 w379 w420] -> w38
      tunnel: [w85 w106 w136 w304 w346 w378 w419] -> w37
      tunnel: w36 -> [w88 w109 w139 w307 w349 w381 _]
      tunnel: w35 -> [w87 w108 w138 w306 w348 w380 _]
      tunnel: w34 -> [w86 w107 w137 w305 w347 w379 _]
      tunnel: w33 -> [w85 w106 w136 w304 w346 w378 _]
      tunnel: [w84 w114 w135 w303 w345 w377 w418] -> w29
      tunnel: w30 -> [w84 w114 w134 w303 w345 w377 w418]
      frame Default {
      }
      frame 69 {
        n11 = Index Array(array=w129, index #1=0 ("index"), index #2=1 ("index")) -> (element #1=w126:u8, element #2=w125:u8)
        n12 = Join Numbers(hi=w126, lo=w125) -> ((hi.lo)=w124:u16)
        n13 = To Double Precision Float(number=w124) -> (double precision float=w123:dbl)
      }
      frame 385 {
        # "Bamocar"
        n14 = Index Array(array=w170, index #1=1 ("index"), index #2=2 ("index"), index #3=0 ("index")) -> (element #1=w167:u8, element #2=w166:u8, element #3=w163:u8)
        n15 = case shown="73" w163 {
          tunnel: w167 -> [_ w184 w201 w226 w238 w249 w270 w286 w296]
          tunnel: w166 -> [_ w185 w200 w225 w237 w250 w269 w285 w295]
          tunnel: [w178 w189 w205 w214 w240 w254 w272 w288 w302] -> w162
          tunnel: w164 -> [w178 w189 w205 _ w240 w254 w272 w288 w302]
          tunnel: [w175 w191 w208 w220 w235 w256 w259 w283 w300] -> w161
          tunnel: [w176 w192 w207 w221 w227 w255 w267 w284 w301] -> w160
          tunnel: [w177 w190 w209 w222 w236 w257 w268 w276 w294] -> w159
          tunnel: w158 -> [w177 w190 w209 w222 w236 w257 w268 _ w294]
          tunnel: w157 -> [w176 w192 w207 w221 _ w255 w267 w284 w301]
          tunnel: w156 -> [w175 w191 w208 w220 w235 w256 _ w283 w300]
          tunnel: [w174 w179 w210 w217 w234 w258 w266 w282 w293] -> w155
          tunnel: w154 -> [w174 _ w210 w217 w234 w258 w266 w282 w293]
          tunnel: [w173 w183 w206 w216 w231 w244 w265 w281 w292] -> w153
          tunnel: w152 -> [w173 w183 w206 w216 w231 _ w265 w281 w291]
          tunnel: [w172 w182 w197 w215 w230 w248 w264 w280 w291] -> w151
          tunnel: w150 -> [w172 w182 _ w215 w230 w248 w264 w280 w292]
          tunnel: [w171 w181 w195 w213 w229 w243 w261 w275 w289] -> w135
          tunnel: w134 -> [w171 w181 w195 w213 w229 w243 w261 w275 _]
          frame 0, Default {
          }
          frame 72 {
            w186 = u8 255 ("x")
            n16 = Subtract(x=w186, y=w185) -> (x-y=w187:u8)
            n17 = Subtract(x=w186, y=w184) -> (x-y=w188:u8)
            n18 = Join Numbers(hi=w187, lo=w188) -> ((hi.lo)=w180:u16)
            n19 = To Double Precision Float(number=w180) -> (double precision float=w179:dbl)
          }
          frame 73 {
            w202 = u8 255 ("x")
            n20 = Subtract(x=w202, y=w200) -> (x-y=w203:u8)
            n21 = Subtract(x=w202, y=w201) -> (x-y=w204:u8)
            n22 = Join Numbers(hi=w203, lo=w204) -> ((hi.lo)=w194:u16)
            n23 = To Double Precision Float(number=w194) -> (double precision float=w193:dbl)
            n24 = Divide(x=w193, y=u16 10000) -> (x/y=w198:dbl)
            n25 = Multiply(x=w198, y=37383.2) -> (x*y=w197:dbl)
          }
          frame 48 {
            w224 = u8 255 ("x")
            n26 = Subtract(x=w224, y=w225) -> (x-y=w219:u8)
            n27 = Subtract(x=w224, y=w226) -> (x-y=w218:u8)
            n28 = Join Numbers(hi=w219, lo=w218) -> ((hi.lo)=w212:u16)
            n29 = To Double Precision Float(number=w212) -> (double precision float=w211:dbl)
            "speed actual" <- w211
            n30 = Divide(x=w211, y=u32 32767) -> (x/y=w214:dbl)
          }
          frame 32 {
            w239 = u8 255 ("x")
            n31 = Subtract(x=w239, y=w237) -> (x-y=w232:u8)
            n32 = Subtract(x=w239, y=w238) -> (x-y=w233:u8)
            n33 = Join Numbers(hi=w232, lo=w233) -> ((hi.lo)=w228:u16)
            n34 = To Double Precision Float(number=w228) -> (double precision float=w227:dbl)
            "Current Actual" <- w227
          }
          frame 95 {
            w251 = u8 255 ("x")
            n35 = Subtract(x=w251, y=w250) -> (x-y=w253:u8)
            n36 = Subtract(x=w251, y=w249) -> (x-y=w252:u8)
            n37 = Join Numbers(hi=w253, lo=w252) -> ((hi.lo)=w242:u16)
            n38 = To Double Precision Float(number=w242) -> (double precision float=w241:dbl)
            n39 = Divide(x=w241, y=u16 10000) -> (x/y=w246:dbl)
            n40 = Multiply(x=w246, y=37383.2) -> (x*y=w244:dbl)
          }
          frame 217 {
            w271 = u8 255 ("x")
            n41 = Subtract(x=w271, y=w269) -> (x-y=w262:u8)
            n42 = Subtract(x=w271, y=w270) -> (x-y=w263:u8)
            n43 = Join Numbers(hi=w262, lo=w263) -> ((hi.lo)=w260:u16)
            n44 = To Double Precision Float(number=w260) -> (double precision float=w259:dbl)
            "Current 200pc" <- w259
          }
          frame 198 {
            w287 = u8 255 ("x")
            n45 = Subtract(x=w287, y=w285) -> (x-y=w278:u8)
            n46 = Subtract(x=w287, y=w286) -> (x-y=w279:u8)
            n47 = Join Numbers(hi=w278, lo=w279) -> ((hi.lo)=w274:u16)
            n48 = To Double Precision Float(number=w274) -> (double precision float=w273:dbl)
            n49 = Divide(x=w273, y=u16 10) -> (x/y=w276:dbl)
            "Current Device" <- w276
          }
          frame 206 {
            w299 = u8 255 ("x")
            n50 = Subtract(x=w299, y=w295) -> (x-y=w298:u8)
            n51 = Subtract(x=w299, y=w296) -> (x-y=w297:u8)
            n52 = Join Numbers(hi=w298, lo=w297) -> ((hi.lo)=w290:u16)
            n53 = To Double Precision Float(number=w290) -> (double precision float=w289:dbl)
          }
        }
      }
      frame 400 {
        w326 = u16 1000 ("y")
        # "AMS 1"
        n54 = Index Array(array=w344, index #1=0 ("index"), index #2=1 ("index"), index #3=2 ("index"), index #4=3 ("index"), index #5=4 ("index"), index #6=5 ("index"), index #7=6 ("index"), index #8=7 ("index")) -> (element #1=w335:u8, element #2=w334:u8, element #3=w333:u8, element #4=w332:u8, element #5=w331:u8, element #6=w330:u8, element #7=w329:u8, element #8=w328:u8)
        n55 = Join Numbers(hi=w334, lo=w335) -> ((hi.lo)=w325:u16)
        n56 = Join Numbers(hi=w330, lo=w331) -> ((hi.lo)=w315:u16)
        n57 = Join Numbers(hi=w328, lo=w329) -> ((hi.lo)=w314:u16)
        n58 = Join Numbers(hi=w332, lo=w333) -> ((hi.lo)=w327:u16)
        n59 = Divide(x=w325, y=w326) -> (x/y=w317:dbl)
        n60 = Divide(x=w327, y=w326) -> (x/y=w316:dbl)
      }
      frame 401 {
        # "AMS 2"
        n61 = Index Array(array=w375, index #1=0 ("index"), index #2=1 ("index"), index #3=2 ("index"), index #4=3 ("index")) -> (element #1=w370:u8, element #2=w369:u8, element #3=w368:u8, element #4=w367:u8)
        n62 = Join Numbers(hi=w369, lo=w370) -> ((hi.lo)=w366:u16)
        n63 = Join Numbers(hi=w367, lo=w368) -> ((hi.lo)=w365:u16)
      }
      frame 600 {
        # "Vector Sensor Data"
        n64 = Index Array(array=w417, index #1=0 ("index"), index #2=1 ("index"), index #3=2 ("index"), index #4=3 ("index"), index #5=4 ("index"), index #6=5 ("index"), index #7=6 ("index"), index #8=7 ("index")) -> (element #1=w408:u8, element #2=w407:u8, element #3=w406:u8, element #4=w405:u8, element #5=w403:u8, element #6=w404:u8, element #7=w402:u8, element #8=w401:u8)
        n65 = Join Numbers(hi=w401, lo=w402) -> ()  [unwired: 1 out]
        n66 = Join Numbers(hi=w407, lo=w408) -> ((hi.lo)=w386:u16)
        n67 = Join Numbers(hi=w405, lo=w406) -> ((hi.lo)=w382:u16)
        n68 = Join Numbers(hi=w404, lo=w403) -> ((hi.lo)=w384:u16)
        n69 = To Double Precision Float(number=w386) -> (double precision float=w387:dbl)
        n70 = To Double Precision Float(number=w382) -> (double precision float=w383:dbl)
        n71 = To Double Precision Float(number=w384) -> (double precision float=w385:dbl)
      }
      frame 601 {
        # "Vector Sensor Data 2"
        n72 = Index Array(array=w443, index #1=0 ("index"), index #2=1 ("index"), index #3=2 ("index"), index #4=3 ("index"), index #5=4 ("index"), index #6=5 ("index"), index #7=6 ("index"), index #8=7 ("index")) -> (element #1=w434:u8, element #2=w433:u8, element #3=w432:u8, element #4=w431:u8, element #5=w430:u8, element #6=w429:u8, element #7=w428:u8, element #8=w427:u8)
        n73 = Join Numbers(hi=w433, lo=w434) -> ((hi.lo)=w426:u16)
        n74 = Join Numbers(hi=w431, lo=w432) -> ((hi.lo)=w425:u16)
        n75 = Join Numbers(hi=w429, lo=w430) -> ((hi.lo)=w424:u16)
        n76 = Join Numbers(hi=w427, lo=w428) -> ((hi.lo)=w423:u16)
        n77 = To Double Precision Float(number=w426) -> (double precision float=w422:dbl)
        n78 = To Double Precision Float(number=w425) -> (double precision float=w421:dbl)
        n79 = To Double Precision Float(number=w424) -> (double precision float=w420:dbl)
        n80 = To Double Precision Float(number=w423) -> (double precision float=w419:dbl)
      }
    }
    "IGBT temp" <- w66
    "I Filter" <- w64
    "Motor Temp" <- w62
    "Highest Cell Volt" <- w57
    "Lowest Cell Volt" <- w58
    "Highest Temp" <- w59
    "Lowest Temp" <- w60
    "Current Sensor" <- w50
    "Accumulator Voltage" <- w52
    "WS FL" <- w48
    "WS FR" <- w46
    "WS RL" <- w45
    "WS RR" <- w44
    "Accelerometer x" <- w44
    "Accelerometer y" <- w40
    "Accelerometer z" <- w39
    "Torque Constant" <- w37
    "Speed Rpm max int" <- w29
    n81 = Divide(x=w70, y=w71) -> (x/y=w76:dbl)
    n82 = Multiply(x=w29, y=w32) -> (x*y=→"Motor RPM":dbl)
    n83 = Multiply(x=w76, y=w72) -> (x*y=w75:dbl)
    n84 = Multiply(x=0.2, y=w75) -> (x*y=→"Actual Bamocar Current":dbl)
    n85 = node-c288() -> ()  [unwired: 1 in, 1 out]
  }
  n86 = timed-loop {
    tunnel: "stop" -> [w506]
    timing: w24 -> [_]
    timing-out: [_] -> w23
    stop <- w506 stop-if-true
    # "If torque constant is NOT BETWEEN 120 and 150, it will be set to 120, to change this, adjust the limits above."
    # "Changes done to apps:\n1) limit set to 35 percent"
    # "To disable power map script, DO NOT DELETE, in last switch case FALSE CASE connect the bottom right square to top left square."
    # "APPS Input - Plausibility Check - APPS Output Command"
    n87 = node-c288() -> ()  [unwired: 1 in, 1 out]
    n88 = xnode "Analog input (1 sample) 2"() -> ("APPS 1 Input (B/AI0 (Pin 3))"=w508:dbl, "APPS 2 Input (B/AI1 (Pin 5))"=w507:dbl)  [unwired: 1 in, 1 out]
    "APPS1 (V) Input (B/AI0 (Pin 3))" <- w508
    "APPS2 (V) Input (B/AI1 (Pin 5))" <- w507
    n89 = Multiply(x=w507, y=1.17857) -> (x*y=w487:dbl)
    "APPS2 Scaled Up (V)" <- w487
    n90 = Multiply(x=w508, y=1.04166) -> (x*y=w465:dbl)
    "APPS1 Scaled Up (V)" <- w465
    n91 = Add(x=w487, y=w465) -> (x+y=w489:dbl)
    n92 = Multiply(x=w465, y=20.0) -> (x*y=w497:dbl)
    n93 = Multiply(x=w465, y=20.0) -> (x*y=w491:dbl)
    "APPS1 %" <- w491
    "APPS1" <- w491
    n94 = Multiply(x=w487, y=30.3) -> (x*y=w464:dbl)
    "APPS2 %" <- w464
    "APPS2" <- w464
    n95 = local read "RTD Brake"() -> (w490:bool)
    n96 = Divide(x=w489, y=2.0) -> ()  [unwired: 1 out]
    n97 = Greater?(x=w497, y=35.0) -> (0:w510:bool)
    n98 = Add(x=w464, y=w465) -> (x+y=w463:dbl)
    n99 = Subtract(x=w464, y=w491) -> (x-y=w525:dbl)
    n100 = Subtract(x=w491, y=w464) -> (x-y=w512:dbl)
    n101 = And(x=w490, y=w510) -> (x .and. y?=w483:bool)
    n102 = Greater?(x=w464, y=175.0) -> (0:w522:bool)
    n103 = Greater?(x=w491, y=175.0) -> (0:w521:bool)
    n104 = case shown="True" w483 {
      tunnel: [FALSE w669] -> w482
      frame False {
      }
      frame True {
        n105 = Tick Count (ms)() -> (millisecond timer value=w671:u32)
        n106 = Greater?(x=w671, y=u32 500) -> (0:w669:bool)
      }
    }
    n107 = Or(x=w522, y=w521) -> (x .or. y?=w520:bool)
    n108 = local read "RTD Buzzer"() -> (w503:bool)
    n109 = Divide(x=w463, y=2.0) -> (x/y=w461:dbl)
    n110 = Greater?(x=w525, y=10.0) -> (0:w526:bool)
    n111 = Greater?(x=w512, y=10.0) -> (0:w513:bool)
    n112 = case shown="False" w503 {
      tunnel: [w718 0] -> w502
      tunnel: w461 -> [w718 _]
      frame False {
      }
      frame True {
      }
    }
    n113 = Or(x=w526, y=w513) -> (x .or. y?=w496:bool)
    n114 = case shown="True" w496 {
      tunnel: [FALSE w715] -> w495
      frame False {
      }
      frame True {
        n115 = Tick Count (ms)() -> (millisecond timer value=w717:u32)
        n116 = Greater?(x=w717, y=u32 100) -> (0:w715:bool)
      }
    }
    n117 = Less?(x=w497, y=25.0) -> (x < y?=w493:bool)
    n118 = xnode "SR Bistable"("reset"=w493, "set"=w482) -> ("output"=w494:bool)  [unwired: 1 in, 1 out]
    n119 = Or(x=w482, y=w494) -> (x .or. y?=w485:bool)
    n120 = Or(x=w520, y=w495) -> (x .or. y?=w486:bool)
    n121 = local read "Torque Constant"() -> (w467:dbl)
    n122 = Or(x=w486, y=w485) -> (x .or. y?=w484:bool)
    "APPS fault" <- w484
    n123 = case shown="False" w484 {
      tunnel: w502 -> [w722 _]
      tunnel: [w722 0.0] -> w501
      frame False {
      }
      frame True {
      }
    }
    "APPS Output (V)" <- w501
    n124 = xnode "LED"("LED0"=w484) -> ()  [unwired: 1 in, 1 out]
    n125 = Greater Or Equal?(x=w467, y=120.0) -> (x >= y?=w469:bool)
    n126 = Less Or Equal?(x=w467, y=150.0) -> (x <= y?=w468:bool)
    n127 = And(x=w469, y=w468) -> (x .and. y?=w470:bool)
    n128 = case shown="True" w470 {
      tunnel: w467 -> [_ w529]
      tunnel: [120.0 ("Torque Constant") w529] -> w466
      frame False {
      }
      frame True {
      }
    }
    n129 = Multiply(x=20, y=w501) -> (x*y=w479:dbl)
    "APPS pedal travel %" <- w479
    n130 = local read "Motor RPM"() -> (w481:dbl)
    n131 = Divide(x=w479, y=100.0) -> (x/y=w478:dbl)
    n132 = Multiply(x=w478, y=w466) -> (x*y=w477:dbl)
    n133 = mathscript code="%Initializing constants\nMax_Power = 80000; %80KW\nefficiency = 0.92; %98% motor and 95% motor controller efficiency\ndouble Motor_Torque_Map;\n\n%Motor RPM saturation\nif RPM >5900\nRPM = 5900\nelseif RPM < 0\nRPM = 0\nelse\nRPM = RPM\nend\n\nMotor_Torque_Map = (Max_Power * 9.550)/(RPM * efficiency); \n%Motor Torque based on 80KW max power\n\nT= min(Motor_Torque_Map, MT); \nTorque = min(T,TC);\n%Outputs minimum of both torques hence limiting the power till 80KW and 200Nm max" "Motor Power Map (80kW)"("MT"=w477, "RPM"=w481, "TC"=w466) -> ("Torque"=w475:dbl)  [unwired: 1 in, 1 out]
    n134 = Divide(x=w475, y=w466) -> (x/y=w474:dbl)
    n135 = Greater?(x=w479, y=100.0) -> (0:w504:bool)
    n136 = Multiply(x=w474, y=5.0) -> (x*y=w473:dbl)
    n137 = case shown="False" w504 {
      tunnel: [w720 5.0 ("APPS output %")] -> w499
      tunnel: w501 -> [_ _]
      tunnel: w473 -> [w720 _]
      frame False {
      }
      frame True {
      }
    }
    n138 = xnode "Analog output (1 sample) 2"("APPS Output (B/AO0 (Pin 2))"=w499) -> ()  [unwired: 1 in, 1 out]
    n139 = Multiply(x=20, y=w499) -> (x*y=→"APPS output %" →"Accelaration":dbl)
    n140 = node-c288() -> ()  [unwired: 1 in, 1 out]
  }
  n141 = timed-loop {
    tunnel: "stop" -> [w843]
    timing: w28 -> [_]
    timing-out: [_] -> w27
    stop <- w843 stop-if-true
    # "Pump Control"
    n142 = node-c288() -> ()  [unwired: 1 in, 1 out]
    n143 = xnode "Digital input (1 sample)"() -> ("B/DIO9 (Pin 29)"=w842:bool)  [unwired: 1 in, 1 out]
    n144 = xnode "Analog input (1 sample)"() -> ("Pump Bamocar (A/AI3 (Pin 9))"=w837:dbl)  [unwired: 1 in, 1 out]
    n145 = xnode "Pulse Timer"("preset time (ms)"=1500, "input"="Pump Test") -> ("output"=w839:bool)  [unwired: 1 in, 2 out]
    n146 = Equal?(x=5.0, y=w837) -> (x = y?=→"Bamocar Temp Threshold":bool)
    n147 = Not(x=w842) -> (.not. x?=w834:bool)
    "Pump out" <- w834
    n148 = Or(x=w834, y=w839) -> (x .or. y?=w838:bool)
    n149 = xnode "Digital output (1 sample)"("Pump out (B/DIO8 (Pin 27))"=w838) -> ()  [unwired: 1 in, 1 out]
    n150 = node-c288() -> ()  [unwired: 1 in, 1 out]
  }
  n151 = timed-loop {
    tunnel: "stop" -> [w1023]
    timing: w26 -> [_]
    timing-out: [_] -> w25
    stop <- w1023 stop-if-true
    # "pin27"
    # "pin25"
    # "Ready-to-Drive Sequence"
    n152 = node-c288() -> ()  [unwired: 1 in, 1 out]
    n153 = xnode "Analog inputs"() -> ("AIR + (B/AI2 (Pin 7))"=w1017:dbl)  [unwired: 1 in, 1 out]
    "AIR +(A9)" <- w1017
    n154 = xnode "Digital input (1 sample) 2"() -> ("RTD Button (B/DIO2 (Pin 15))"=w1016:bool, "RTD Brake (B/DIO3 (Pin 17))"=w1015:bool)  [unwired: 1 in, 1 out]
    n155 = Not(x=w1015) -> (.not. x?=w1009:bool)
    n156 = Divide(x=w1017, y=5.0) -> (x/y=w1021:dbl)
    n157 = Not(x=w1016) -> (.not. x?=w1013:bool)
    "RTD Button" <- w1013
    n158 = local write "RTD Button"(w1013) -> ()
    n159 = Or(x="RTD Brake Test", y=w1009) -> (x .or. y?=w1008:bool)
    "RTD Brake" <- w1008
    n160 = Number To Boolean Array(number=w1021) -> (Boolean array=w1022:bool[])
    n161 = And(x=w1013, y=w1008) -> (x .and. y?=w1018:bool)
    n162 = Not(x="RFE  Test") -> (.not. x?=w995:bool)
    n163 = Index Array(array=w1022, index=0) -> (element=w1007:bool)
    "AIR + Boolean" <- w1007
    n164 = xnode "Pulse Timer"("preset time (ms)"=1500, "input"="EN Test") -> ("output"=w1003:bool)  [unwired: 1 in, 2 out]
    n165 = Or(x=w995, y=w1007) -> (x .or. y?=w1006:bool)
    "RFE Indicator" <- w1006
    n166 = Not(x=w1007) -> (.not. x?=w1011:bool)
    n167 = And(x=w1007, y=w1018) -> (x .and. y?=w1012:bool)
    "RTD Status LED" <- w1012
    n168 = xnode "Digital output (1 sample) 3"("RFE (B/DIO0 (Pin 11))"=w1006) -> ()  [unwired: 1 in, 1 out]
    n169 = xnode "SR Bistable"("reset"=w1011, "set"=w1012) -> ("output"=w1000:bool)  [unwired: 1 in, 1 out]
    n170 = local write "RTD Brake"(w1008) -> ()
    n171 = xnode "Pulse Timer"("preset time (ms)"=1500, "input"=w1000) -> ("output"=w998:bool)  [unwired: 1 in, 2 out]
    n172 = Or(x=w1000, y=w1003) -> (x .or. y?=w1002:bool)
    "EN Indicator" <- w1002
    n173 = xnode "Digital output (1 sample) 2"("EN (B/DIO1 (Pin 13))"=w1002) -> ()  [unwired: 1 in, 1 out]
    n174 = Or(x=w998, y="Buzzer test") -> (x .or. y?=w997:bool)
    "RTD Buzzer" <- w997
    n175 = case shown="True" w997 {
      tunnel: [0.0 ("y") 5.0 ("y")] -> w1014
      frame False {
      }
      frame True {
      }
    }
    n176 = xnode "Analog output (1 sample)"("RTD - Buzzer (B/AO1 (Pin 4))"=w1014) -> ()  [unwired: 1 in, 1 out]
    n177 = node-c288() -> ()  [unwired: 1 in, 1 out]
  }
  n178 = timed-loop {
    tunnel: "stop" -> [w1337]
    timing: w22 -> [_]
    timing-out: [_] -> w21
    stop <- w1337 stop-if-true
    w1370 = 9  # array no.
    # "I2C BMS Data Logging"
    n179 = node-c288() -> ()  [unwired: 1 in, 1 out]
    n180 = local read "Values"() -> (w1368:dbl[])
    "Values" <- w1368
    n181 = local read "Array"() -> (→"Array":u8[])
    n182 = for {
      N: w1370 -> [_]
      shift-right: [w1395] -> _
      shift-left: u8[] [] -> [w1396]
      i -> [w1391]
      w1390 = u32 32 ("Byte Count")
      w1392 = u8 0 ("Slave Address (7-bit)")
      n183 = call "Wait"("Count(uSec)"=u32 20000 ("milliseconds to wait")) -> ()  [unwired: 1 out]
      n184 = Build Array(w1391) -> (w1394:i32[])
      n185 = xnode "I2C"("Slave Address (7-bit)"=w1392, "Bytes to Write"=w1394, "Byte Count"=w1390) -> ("Bytes Read"=w1397:u8[])  [unwired: 1 in, 1 out]
      "Bytes Read" <- w1397
      n186 = Insert Into Array(array=w1396, new element=w1397) -> (w1395:u8[])  [unwired: 1 in]
      n187 = local write "Array"(w1395) -> ()
      "loop counter" <- w1391
      "Slave Address (7-bit)" <- w1392
      "Byte Count" <- w1390
    }
    n188 = Multiply(x=16 ("y"), y=w1370) -> (x*y=w1373:i32)
    n189 = Split 1D Array(array=w1368, index=17) -> (first subarray=→"Stack 1 vol":dbl[], second subarray=w1365:dbl[])
    n190 = for {
      N: w1373 -> [_]
      shift-right: [w1380] -> _
      shift-left: dbl[] [] -> [w1385]
      i -> [w1378]
      n191 = Multiply(x=w1378, y=2 ("x")) -> (x*y=w1388:i32)
      n192 = call "Wait2"("Count(uSec)"=u32 1420) -> ()  [unwired: 1 out]
      n193 = Increment(x=w1388) -> (x+1=w1389:i32)
      n194 = local read "Array"() -> (w1382:u8[])
      n195 = Index Array(array=w1382, index #1=w1388, index #2=w1389) -> (element #1=w1387:u8, element #2=w1386:u8)
      "high byte" <- w1387
      "low byte" <- w1386
      n196 = Join Numbers(hi=w1387, lo=w1386) -> ((hi.lo)=w1384:u16)
      n197 = Divide(x=w1384, y=u16 1000) -> (x/y=w1381:dbl)
      n198 = Insert Into Array(array=w1385, new element=w1381) -> (w1380:dbl[])  [unwired: 1 in]
      n199 = local write "Values"(w1380) -> ()
    }
    n200 = Split 1D Array(array=w1365, index=17) -> (first subarray=→"Stack 2 vol":dbl[], second subarray=w1364:dbl[])
    n201 = Split 1D Array(array=w1364, index=17) -> (first subarray=→"Stack 3 vol":dbl[], second subarray=w1363:dbl[])
    n202 = Split 1D Array(array=w1363, index=17) -> (first subarray=→"Stack 4 vol":dbl[], second subarray=w1362:dbl[])
    n203 = Split 1D Array(array=w1362, index=17) -> (first subarray=→"Stack 5 vol":dbl[], second subarray=w1336:dbl[])
    n204 = Split 1D Array(array=w1336, index=9) -> (first subarray=→"Stack 1 temp":dbl[], second subarray=w1351:dbl[])
    n205 = Split 1D Array(array=w1351, index=9) -> (first subarray=→"Stack 2 temp":dbl[], second subarray=w1350:dbl[])
    n206 = Split 1D Array(array=w1350, index=9) -> (first subarray=→"Stack 3 temp":dbl[], second subarray=w1347:dbl[])
    n207 = Split 1D Array(array=w1347, index=9) -> (first subarray=→"Stack 4 temp":dbl[], second subarray=w1346:dbl[])
    n208 = Split 1D Array(array=w1346, index=9) -> (first subarray=→"Stack 5 temp":dbl[], second subarray=w1335:dbl[])
    n209 = Split 1D Array(array=w1335, index=1) -> (first subarray=→"AMS current":dbl[], second subarray=→"Coulomb Counting":dbl[])
    n210 = node-c288() -> ()  [unwired: 1 in, 1 out]
  }
  n211 = To Double Precision Float(number=u32 1000) -> (double precision float=w7:dbl)
  n212 = To Double Precision Float(number=50.0) -> (double precision float=w9:dbl)
  n213 = Divide(x=w7, y=w9) -> (x/y=w14:dbl)
  n214 = call <vilib>:"Create X-CAN Session.vi"("error in (no error)"=errorcluster {"status"=FALSE, "code"=0, "source"=""}, "CAN Speed [Kbps]"=w4, "MXP Channel"=MXPChannel."A/MXP") -> ("error out"=w6:errorcluster, "X-CAN Session out"=w2:refnum<class "X-CAN.lvclass">)  [unwired: 7 in]
  n215 = To Quad Integer(1:w14) -> (0:w13:i64)
  n216 = node-c288(w27) -> ()  [unwired: 1 out]
  n217 = node-c288(w13) -> (w17:T4)
  n218 = timed-loop "Timed Loop" {
    timing: w17 -> [_]
    timing-out: [_] -> w16
    tunnel: w6 -> [w1439]
    shift-right: [w1454] -> w11
    shift-left: w2 -> [w1440]
    tunnel: [w1453] -> w12
    shift-right: [w1442] -> _
    shift-left: bool[] [TRUE, FALSE] -> [w1443]
    stop <- w1458 stop-if-true
    # "5."
    # "X-CAN Read"
    n219 = call <vilib>:"Read X-CAN Frame.vi"("error in"=w1439, "X-CAN Session in"=w1440) -> ("error out"=w1448:errorcluster, "CAN Frame"=w1444:T1, "X-CAN Session out"=w1447:refnum<class "X-CAN.lvclass">)  [unwired: 7 in]
    n220 = Unbundle By Name(w1448) -> ("code"=w1449:i32)
    n221 = case shown="8001" w1449 {
      tunnel: w1448 -> [w1465 w1470 w1474]
      tunnel: w1447 -> [w1464 w1468 w1475]
      tunnel: [w1464 w1468 w1475] -> w1459
      tunnel: [w1465 w1469 w1474] -> w1446
      tunnel: [TRUE FALSE _] -> w1445
      tunnel: w1444 -> [w1462 _ _]
      tunnel: [w1462 T1 {"identifier"=0, "extended?"=FALSE, "echo?"=FALSE, "payload"=[], "timestamp"=timestamp(0 s since 1904-01-01)} ("CAN Frame") T1 {"identifier"=0, "extended?"=FALSE, "echo?"=FALSE, "payload"=[], "timestamp"=timestamp(0 s since 1904-01-01)} ("CAN Frame")] -> w1441
      tunnel: w1443 -> [w1461 w1467 w1473]
      tunnel: [w1460 w1467 w1473] -> w1442
      frame 0 {
        n222 = Not(x=w1461) -> (.not. x?=w1460:bool[])
      }
      frame 8001 {
        n223 = call <vilib>:"Clear Errors.vi"("error in (no error)"=w1470) -> ("error out"=w1469:errorcluster)  [unwired: 5 in, 1 out]
      }
      frame Default {
      }
    }
    "LEDs" <- w1442
    "Data Ready?" <- w1445
    "CAN Frame" <- w1441
    n224 = To Double Precision Float(number=u32 1000) -> (double precision float=w1450:dbl)
    n225 = call <vilib>:"LED_Write.vi"("error in"=w1446, "LED Values"=w1442, "X-CAN in"=w1459) -> ("error out"=w1453:errorcluster, "X-CAN out"=w1454:refnum<class "X-CAN.lvclass">)  [unwired: 7 in]
    n226 = To Double Precision Float(number=50.0) -> (double precision float=w1451:dbl)
    n227 = Or(x=w1453, y="Stop Button") -> (x .or. y?=w1458:bool)
    n228 = Divide(x=w1450, y=w1451) -> (x/y=w1456:dbl)
    n229 = To Quad Integer(1:w1456) -> (0:w1455:i64)
    n230 = node-c288(w1455) -> ()  [unwired: 1 out]
  }
  n231 = node-c288(w19) -> ()  [unwired: 1 out]
  n232 = node-c288(w16) -> ()  [unwired: 1 out]
  n233 = call <vilib>:"Clear X-CAN Session.vi"("error in (no error)"=w12, "X-CAN Session in"=w11) -> ("error out"=w10:errorcluster)  [unwired: 9 in]
  n234 = node-c288(w25) -> ()  [unwired: 1 out]
  n235 = call <vilib>:"Simple Error Handler.vi"("error in (no error)"=w10) -> ()  [unwired: 4 in, 5 out]
  n236 = node-c288(w21) -> ()  [unwired: 1 out]
  n237 = node-c288(w23) -> ()  [unwired: 1 out]
